vi "Symphony Read Det Uniq_ID.vi"(8 "error in (no error)":errorcluster) -> (0 "error out":errorcluster, 1 "Name":string[](array[string]), 2 "DeviceName":string[](array[string]), 3 "UniqueID":string[](array[string]), 4 "nbr of components":i32)   [LabVIEW 2019]
uses:
  <vilib>/registry/registry.llb/Registry SAM.ctl
  <vilib>/registry/registry.llb/Registry RtKey.ctl
  <vilib>/registry/registry.llb/Read Registry Value Simple STR.vi
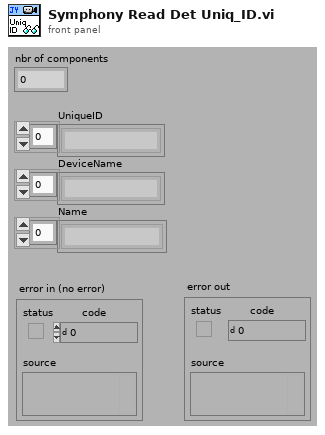
[diagram p1: front panel]
types:
  T1 = enum16{"ReadRegKeys", "GetCCDKeys", "ReadKeyData", "Error"}
  T2 = typedef "Registry SAM.ctl" = enum32{"KEY_QUERY_VALUE", "KEY_SET_VALUE", "KEY_CREATE_SUB_KEY", "KEY_ENUMERATE_SUB_KEYS", "KEY_NOTIFY", "KEY_CREATE_LINK", "KEY_READ", "KEY_WRITE", "KEY_ALL_ACCESS", "KEY_READ | KEY_WRITE"}
  T3 = typedef "Registry RtKey.ctl" = enum32{"HKEY_CLASSES_ROOT", "HKEY_CURRENT_USER", "HKEY_LOCAL_MACHINE", "HKEY_USERS", "HKEY_PERFORMANCE_DATA", "HKEY_CURRENT_CONFIG", "HKEY_DYN_DATA"}
  T4 = typedef "Registry refnum.ctl" = refnum<k1>
  T5 = cluster{"numSubKeys":i32, "maxSubKeyLen":i32, "maxSubKeyClassLen":i32}
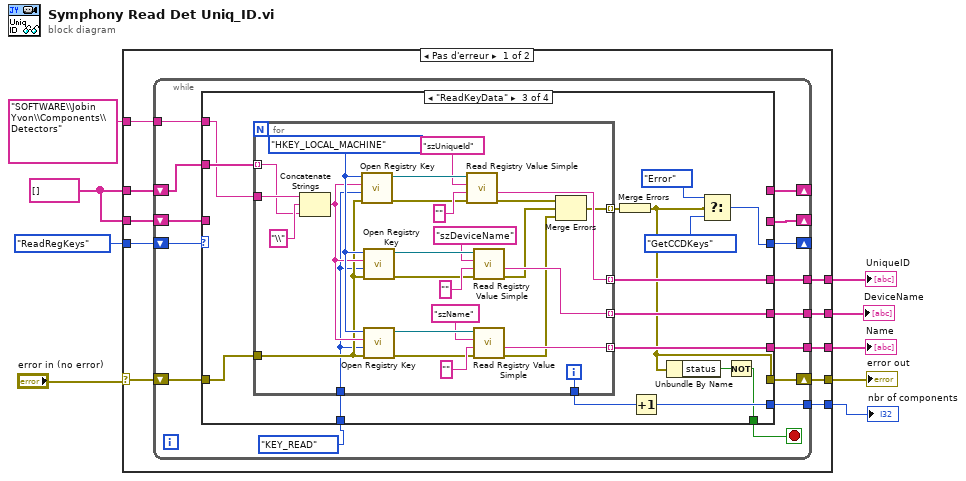
[diagram p0: block diagram]
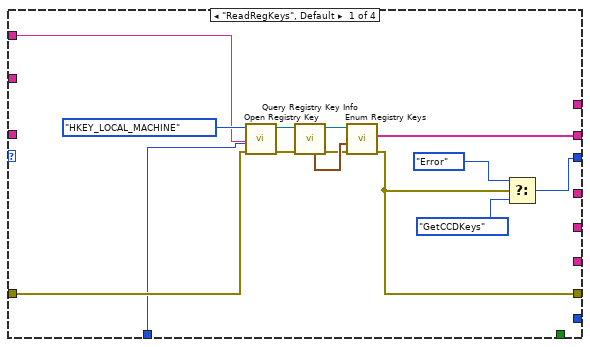
[diagram p2: hidden frame]
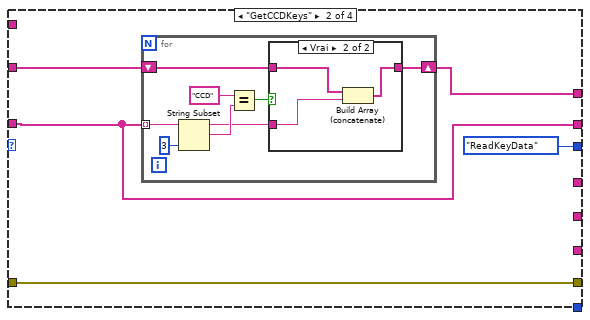
[diagram p3: hidden frame]
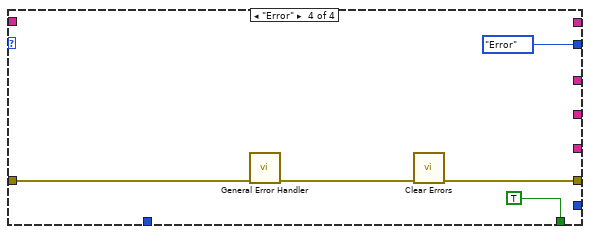
[diagram p5: hidden frame]
diagram:
  w7 = string[] [] ("test")
  n1 = case shown="Pas d'erreur" "error in (no error)" {
    selector: "error in (no error)" -> [w17 w113]
    tunnel: T1."ReadRegKeys" -> [w19 _]
    tunnel: w7 -> [w18 _]
    tunnel: w7 -> [w16 _]
    tunnel: [w15 _] -> w6
    tunnel: [w14 w113] -> w5
    tunnel: [w13 _] -> w4
    tunnel: [w12 _] -> w3
    tunnel: [w11 _] -> w2
    tunnel: "SOFTWARE\\Jobin Yvon\\Components\\Detectors" ("subkey") -> [w10 _]
    frame No Error {
      n2 = while {
        shift-right: [w26] -> _
        shift-left: w19 -> [w33]
        shift-right: [w29] -> _
        shift-left: w18 -> [w32]
        shift-right: [w28] -> w14
        shift-left: w17 -> [w34]
        shift-right: [w31] -> _
        shift-left: w16 -> [w30]
        tunnel: [w27] -> w15
        tunnel: [w25] -> w13
        tunnel: [w24] -> w12
        tunnel: [w23] -> w11
        tunnel: w10 -> [w21]
        stop <- w22 stop-if-true
        n3 = case shown="\"ReadKeyData\"" w33 {
          tunnel: w34 -> [w41 w49 w80 w111]
          tunnel: w32 -> [_ w53 w77 _]
          tunnel: [w42 w51 _ _] -> w31
          tunnel: w30 -> [_ w51 _ _]
          tunnel: [_ w52 _ _] -> w29
          tunnel: [w40 w49 w69 w109] -> w28
          tunnel: [_ _ w78 _] -> w27
          tunnel: [w37 T1."ReadKeyData" w72 T1."Error"] -> w26
          tunnel: [_ _ w75 _] -> w25
          tunnel: [_ _ w71 _] -> w24
          tunnel: [_ _ w70 _] -> w23
          tunnel: [_ _ w67 TRUE] -> w22
          tunnel: w21 -> [w36 _ w66 _]
          tunnel: Registry_SAM."KEY_READ" ("security access mask (KEY_READ | KEY_WRITE)") -> [w35 _ w65 _]
          frame "ReadRegKeys", Default {
            n4 = call <vilib>:"Open Registry Key.vi"("error in (no error)"=w41, "security access mask (KEY_READ | KEY_WRITE)"=w35, "subkey"=w36, "root key (HKEY_LOCAL_MACHINE)"=Registry_RtKey."HKEY_LOCAL_MACHINE") -> ("error out"=w46:errorcluster, "refnum out"=w47:T4)  [unwired: 6 in]
            n5 = call <vilib>:"Query Registry Key Info.vi"("error in (no error)"=w46, "refnum"=w47) -> ("error out"=w44:errorcluster, "refnum out"=w43:T4, "subkey info"=w48:T5)  [unwired: 5 in, 2 out]
            n6 = call <vilib>:"Enum Registry Keys.vi"("error in (no error)"=w44, "subkey info"=w48, "refnum"=w43) -> ("error out"=w40:errorcluster, "subkeys"=w42:string[])  [unwired: 6 in, 1 out]
            n7 = Select(t=T1."Error", s=w40, f=T1."GetCCDKeys") -> (s? t:f=w37:T1)
          }
          frame "GetCCDKeys" {
            n8 = for {
              tunnel: w51 -> [w56] mode=indexing
              shift-right: [w54] -> w52
              shift-left: w53 -> [w55]
              n9 = String Subset(string=w56, length (rest)=3 ("longueur (reste)")) -> (substring=w57:string)  [unwired: 1 in]
              n10 = Equal?(x="CCD", y=w57) -> (x = y?=w58:bool)
              n11 = case shown="Vrai" w58 {
                tunnel: w56 -> [_ w64]
                tunnel: w55 -> [w61 w63]
                tunnel: [w61 w62] -> w54
                frame False {
                }
                frame True {
                  n12 = Build Array (concatenate)(w63, w64) -> (w62:string[])
                }
              }
            }
          }
          frame "ReadKeyData" {
            n13 = for {
              tunnel: w77 -> [w87] mode=indexing
              tunnel: w66 -> [w105]
              tunnel: [w106] -> w78 mode=indexing
              tunnel: [w92] -> w71 mode=indexing
              tunnel: [w91] -> w70 mode=indexing
              tunnel: [w90] -> w76
              tunnel: w80 -> [w86]
              tunnel: [w82] -> w79 mode=indexing
              tunnel: w65 -> [w81]
              i -> [w90]
              w93 = Registry_RtKey."HKEY_LOCAL_MACHINE" ("root key (HKEY_LOCAL_MACHINE)")
              n14 = Concatenate Strings(w105, "\\" ("Sous-chaîne"), w87) -> (w89:string)
              n15 = call <vilib>:"Open Registry Key.vi"("error in (no error)"=w86, "security access mask (KEY_READ | KEY_WRITE)"=w81, "subkey"=w89, "root key (HKEY_LOCAL_MACHINE)"=w93) -> ("error out"=w103:errorcluster, "refnum out"=w104:T4)  [unwired: 6 in]
              n16 = call <vilib>:"Open Registry Key.vi"("error in (no error)"=w86, "security access mask (KEY_READ | KEY_WRITE)"=w81, "subkey"=w89, "root key (HKEY_LOCAL_MACHINE)"=w93) -> ("error out"=w99:errorcluster, "refnum out"=w100:T4)  [unwired: 6 in]
              n17 = call <vilib>:"Open Registry Key.vi"("error in (no error)"=w86, "security access mask (KEY_READ | KEY_WRITE)"=w81, "subkey"=w89, "root key (HKEY_LOCAL_MACHINE)"=w93) -> ("error out"=w95:errorcluster, "refnum out"=w96:T4)  [unwired: 6 in]
              n18 = call-poly <vilib>:"Read Registry Value Simple.vi"("error in (no error)"=w103, "default data"="", "value"="szUniqueId" ("Sous-chaîne"), "refnum"=w104) -> ("error out"=w85:errorcluster, "String/Binary data"=w106:string)  [unwired: 2 in, 2 out]
              n19 = call-poly <vilib>:"Read Registry Value Simple.vi"("error in (no error)"=w99, "default data"="", "value"="szDeviceName", "refnum"=w100) -> ("error out"=w84:errorcluster, "String/Binary data"=w92:string)  [unwired: 2 in, 2 out]
              n20 = call-poly <vilib>:"Read Registry Value Simple.vi"("error in (no error)"=w95, "default data"="", "value"="szName", "refnum"=w96) -> ("error out"=w83:errorcluster, "String/Binary data"=w91:string)  [unwired: 2 in, 2 out]
              n21 = Merge Errors(w85, w84, w83) -> (w82:errorcluster)
            }
            n22 = Merge Errors(w79) -> (w69:errorcluster)
            n23 = Increment(x=w76) -> (x+1=w75:i32)
            n24 = Unbundle By Name(w69) -> ("status"=w68:bool)
            n25 = Select(t=T1."Error", s=w69, f=T1."GetCCDKeys") -> (s? t:f=w72:T1)
            n26 = Not(x=w68) -> (.not. x?=w67:bool)
          }
          frame "Error" {
            n27 = call <vilib>:"General Error Handler.vi"("error in (no error)"=w111) -> ("error out"=w110:errorcluster)  [unwired: 10 in, 4 out]
            n28 = call <vilib>:"Clear Errors.vi"("error in (no error)"=w110) -> ("error out"=w109:errorcluster)  [unwired: 5 in, 1 out]
          }
        }
      }
    }
    frame Error {
    }
  }
  "error out" <- w5
  "Name" <- w2
  "DeviceName" <- w3
  "UniqueID" <- w6
  "nbr of components" <- w4
